vi "GetID.vi"(8 "error in (no error)":errorcluster) -> (0 "error out":errorcluster, 2 "Computer ID":string)   [LabVIEW 2019, in "Tools.lvlib"]
uses:
  Tools.lvlib
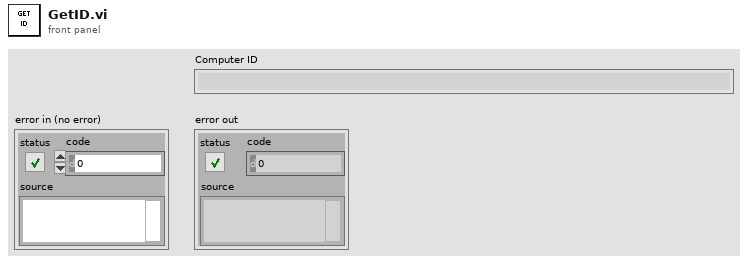
[diagram p1: front panel]
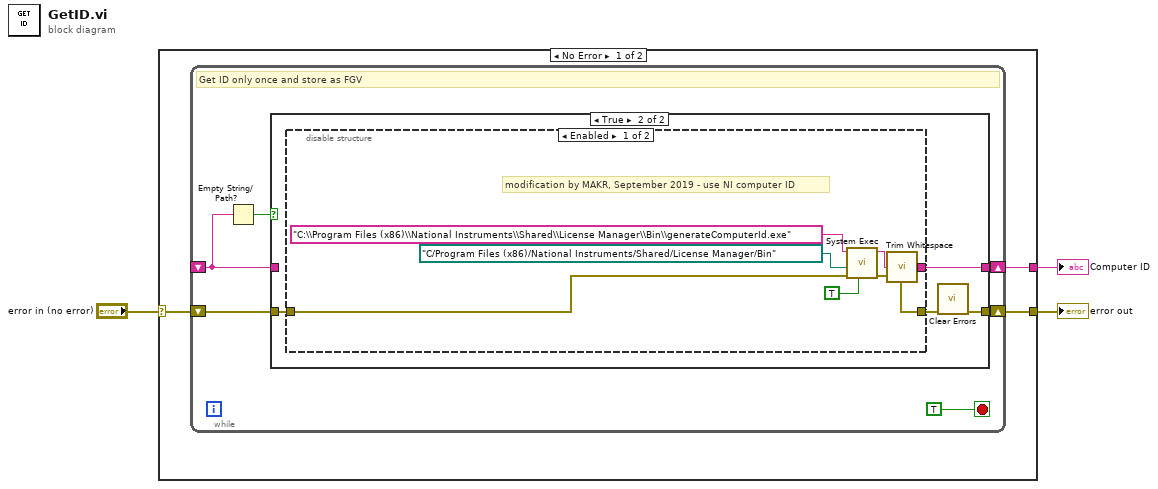
[diagram p0: block diagram]
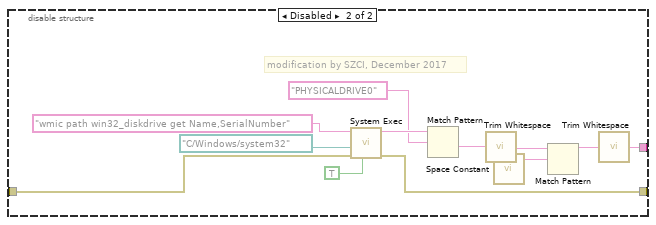
[diagram p3: hidden frame]
diagram:
  n1 = case shown="No Error" "error in (no error)" {
    selector: "error in (no error)" -> [w5 w38]
    tunnel: [w6 _] -> w3
    tunnel: [w4 w38] -> w1
    frame No Error {
      n2 = while {
        shift-right: [w10] -> w4
        shift-left: w5 -> [w12]
        shift-right: [w11] -> w6
        shift-left: _ -> [w7]
        stop <- TRUE stop-if-true
        # "Get ID only once and store as FGV"
        n3 = Empty String/Path?(string/path=w7) -> (empty?=w8:bool)
        n4 = case shown="True" w8 {
          tunnel: w12 -> [w13 w18]
          tunnel: [w14 w17] -> w11
          tunnel: [w13 w15] -> w10
          tunnel: w7 -> [w14 _]
          frame False {
          }
          frame True {
            n5 = disable-structure shown="Enabled" {
              disable-tunnel: w18 -> [w22 w34]
              disable-tunnel: [w19 w27] -> w17
              disable-tunnel: [w20 w26] -> w16
              frame Enabled {
                # "modification by MAKR, September 2019 - use NI computer ID"
                n6 = call <vilib>:"System Exec.vi"("run minimized? (F)"=TRUE, "error in (no error)"=w22, "working directory"=path "C:/Program Files (x86)/National Instruments/Shared/License Manager/Bin", "command line"="C:\\Program Files (x86)\\National Instruments\\Shared\\License Manager\\Bin\\generateComputerId.exe") -> ("error out"=w20:errorcluster, "standard output"=w21:string)  [unwired: 4 in, 2 out]
                n7 = call <vilib>:"Trim Whitespace.vi"("string"=w21) -> ("trimmed string"=w19:string)  [unwired: 1 in]
              }
              frame Disabled {
                # "modification by SZCI, December 2017"
                n8 = call <vilib>:"System Exec.vi"("run minimized? (F)"=TRUE, "error in (no error)"=w34, "working directory"=path "C:/Windows/system32", "command line"="wmic path win32_diskdrive get Name,SerialNumber") -> ("error out"=w26:errorcluster, "standard output"=w33:string)  [unwired: 4 in, 2 out]
                n9 = Match Pattern(string=w33, regular expression="PHYSICALDRIVE0") -> (after substring=w31:string)  [unwired: 1 in, 3 out]
                n10 = call <vilib>:"Trim Whitespace.vi"("string"=w31) -> ("trimmed string"=w30:string)  [unwired: 1 in]
                n11 = call <vilib>:"Space Constant.vi"() -> ("String"=w29:string)
                n12 = Match Pattern(string=w30, regular expression=w29) -> (before substring=w28:string)  [unwired: 1 in, 3 out]
                n13 = call <vilib>:"Trim Whitespace.vi"("string"=w28) -> ("trimmed string"=w27:string)  [unwired: 1 in]
              }
            }
            n14 = call <vilib>:"Clear Errors.vi"("error in (no error)"=w16) -> ("error out"=w15:errorcluster)  [unwired: 5 in, 1 out]
          }
        }
      }
    }
    frame Error {
    }
  }
  "Computer ID" <- w3
  "error out" <- w1
